vi "Logout.vi"(7 "error in (no error)":errorcluster, 10 "reference in":refnum<class "MES_Local.lvclass">) -> (0 "error out":errorcluster, 3 "reference in":refnum<class "MES_Local.lvclass">)   [LabVIEW 2022 SP3, in "MES_Local.lvlib" / "MES_Local.lvclass"]
uses:
  MES_Local.lvclass
  Components/Login_Base.lvlibp/Login_Base.lvclass
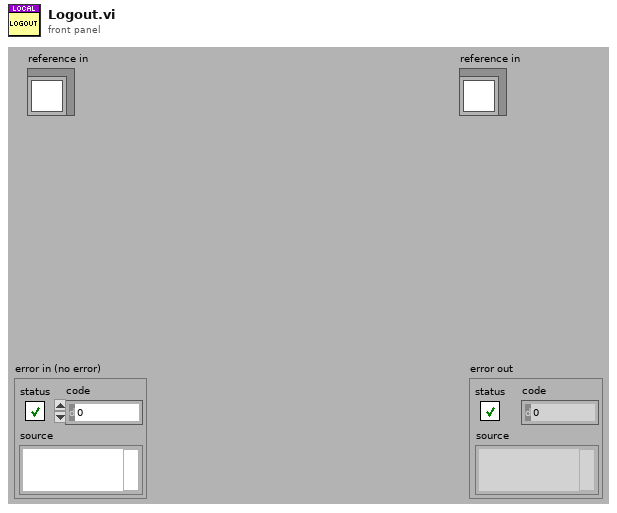
[diagram p1: front panel]
types:
  T1 = typedef "MES_Local.lvlib/MES_Local.lvclass/ObjectAttributes.ctl" = cluster{"Config":T2, "Logged_In?":bool, "AttributeNames":string[], "AttributeWritten":bool[], "ComponentNames":string[], "TestIndex":i32, "TestTag":string[], "Time Stamp":timestamp, "Employee":string, "Resource_Key":string, "Local Spec":path, "Login":refnum<class "Login_Base.lvclass">, "ReportPath":path, "Spec":T3, "StartTime":timestamp, "Role":string}
  T2 = typedef "MES_Local.lvlib/MES_Local.lvclass/Config.ctl" = cluster{"Results_Path":path}
  T3 = typedef "MES_Base.lvlibp/MES_Base.lvclass/Spec.ctl" = cluster{"Header":cluster{"Doctype":string, "Checksum":string, "DriverKey":string, "SpecId":string, "TransactionId":string, "AccountId":string, "SpecName":string, "WorkflowStep":string, "SerialNumber":string, "BatchNumber":string, "Status":enum16{"Pending", "Pass", "Fail"}, "Comment":string, "FirstFail":string, "Employee":string, "LocalMachine":string, "ResourceKey":string, "Date":string, "Time":string, "Duration":string, "DUT Position":i32}, "Components":cluster{"SerialNumber":string, "PartNumber":string, "Revision":string, "BatchNumber":string, "Name":string, "Description":string, "Attached":bool}[], "Attributes":cluster{"Name":string, "Description":string, "DataType":enum16{"NA", "String", "Boolean", "Int", "Dbl"}, "Value":variant, "DisplayFormat":string, "ReadOnly":bool, "Required":bool}[], "Tests":cluster{"Code":string, "Name":string, "Description":string, "Group":string, "IsGroup":bool, "Tag":string, "Method":string, "Parrameter":string, "DataType":enum16{"NA", "String", "Boolean", "Int", "Dbl"}, "Value":variant, "Status":enum16{"Pending", "Pass", "Fail"}, "LimitLo":variant, "LimitHi":variant, "StringMatch":string, "BooleanMatch":bool, "DisplayFormat":string, "Units":string, "TestTime":dbl}[]}
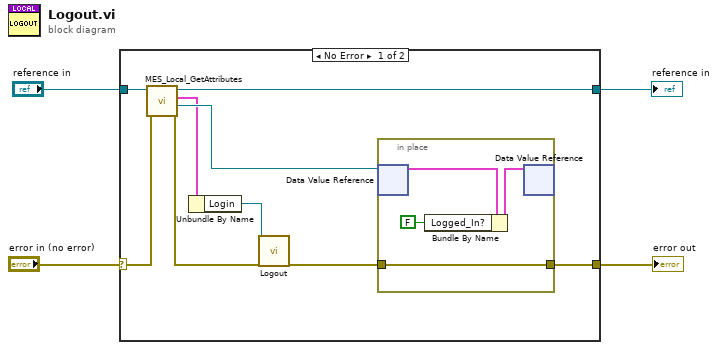
[diagram p0: block diagram]
diagram:
  n1 = case shown="No Error" "error in (no error)" {
    selector: "error in (no error)" -> [w13 w19]
    tunnel: [w5 w19] -> w3
    tunnel: [w11 w18] -> w1
    tunnel: "reference in" -> [w12 w18]
    frame No Error {
      n2 = call "MES_Local_GetAttributes.vi"("error in (no error)"=w13, "reference in"=w12) -> ("error out"=w9:errorcluster, "DataRef"=w10:refnum<data-value>, "Data"=w8:T1, "reference out"=w11:refnum<class "MES_Local.lvclass">)  [unwired: 6 in]
      n3 = Unbundle By Name(w8) -> ("Login"=w7:refnum<class "Login_Base.lvclass">)
      n4 = call-dynamic "Logout.vi"("reference in"=w7, "error in (no error)"=w9) -> ("error out"=w6:errorcluster)  [unwired: 16 in, 1 out]
      n5 = in-place {
        in-place-border: w6 -> [w14]
        in-place-border: [w14] -> w5
        n6 = in-place-dvr #1(w10) -> (w17:T1)  [unwired: 1 out]
        n7 = Bundle By Name(cluster=w17, "Logged_In?"=FALSE) -> (w16:T1)
        n8 = in-place-dvr #1(w16) -> ()  [unwired: 2 out]
      }
    }
    frame Error {
    }
  }
  "error out" <- w3
  "reference in" <- w1
